vi "NI VeriStand - Close Alarm Manager Reference.vi"(8 "error in (no error)":errorcluster, 11 "AlarmManager":T1) -> (0 "error out":errorcluster)   [LabVIEW 2020, in "NI_VS AlarmManager ExecutionAPI.lvlib"]
doc: "Closes an open reference to the alarm manager on the VeriStand Gateway. Use this VI to close each alarm manager reference that you open with the Open Alarm Manager Reference VI."
uses:
  <vilib>/NI VeriStand/Execution/AlarmManager/NI_VS AlarmManager ExecutionAPI.lvlib
  <vilib>/NI VeriStand/Execution/AlarmManager/AlarmManagerAPI.ctl
  NationalInstruments.VeriStand.ClientAPI
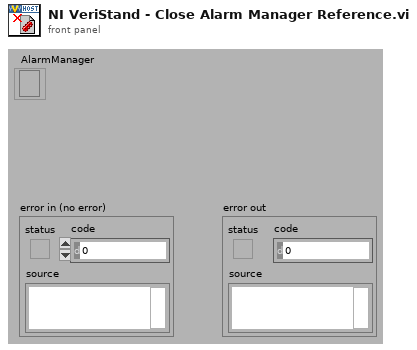
[diagram p1: front panel]
types:
  T1 = typedef "NI_VS AlarmManager ExecutionAPI.lvlib/AlarmManagerAPI.ctl" = refnum<k24>
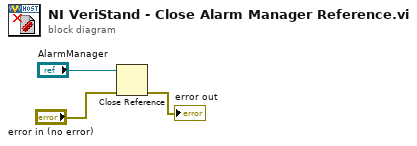
[diagram p0: block diagram]
diagram:
  n1 = Close Reference(reference="AlarmManager", error in (no error)="error in (no error)") -> (error out=→"error out":errorcluster)
